vi "Read Controls.vi"(8 "Error In":errorcluster, 10 "Digital Input Task In":refnum<k21>, 11 "Analog Input Task In":refnum<k21>) -> (0 "Error Out":errorcluster, 1 "Octave Out":bool, 2 "Harmony Out":bool, 3 "Analog Input Task Out":refnum<k21>, 5 "Volume Out":dbl)   [LabVIEW 2020]
doc: "Read Controls.vi reads the voltage across the potentiometer and the state of the two digital buttons to determine the Volume double-precision floating-point value and the digital Harmony and Octave Boolean values."
uses:
  <vilib>/DAQmx/read.llb/DAQmx Read (Analog 1D DBL NChan 1Samp).vi
  <vilib>/DAQmx/read.llb/DAQmx Read (Digital 1D Bool 1Chan 1Samp).vi
  <vilib>/DAQmx/miscellaneous.llb/DAQmx Fill In Error Info.vi
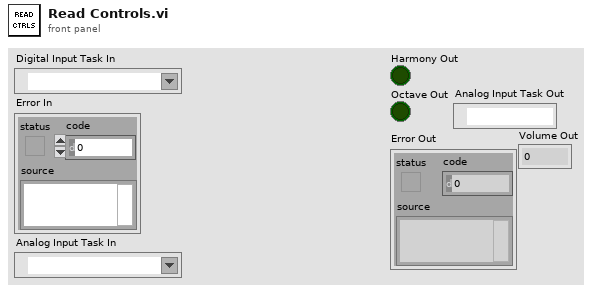
[diagram p1: front panel]
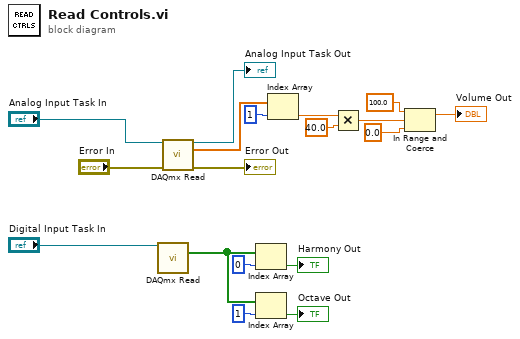
[diagram p0: block diagram]
diagram:
  n1 = call-poly <vilib>:"DAQmx Read.vi"("task/channels in"="Digital Input Task In") -> ("data"=w17:bool[])  [unwired: 12 in, 2 out]
  n2 = call-poly <vilib>:"DAQmx Read.vi"("task/channels in"="Analog Input Task In", "error in"="Error In") -> ("task out"=→"Analog Input Task Out":refnum<k21>, "data"=w13:dbl[], "error out"=→"Error Out":errorcluster)  [unwired: 11 in]
  n3 = Index Array(array=w17, index=0) -> (element=→"Harmony Out":bool)
  n4 = Index Array(array=w17, index=1) -> (element=→"Octave Out":bool)
  n5 = Index Array(array=w13, index=1) -> (element=w12:dbl)
  n6 = Multiply(x=w12, y=40.0) -> (x*y=w7:dbl)
  n7 = In Range and Coerce(upper limit=100.0, x=w7, lower limit=0.0) -> (coerced(x)=→"Volume Out":dbl)  [unwired: 1 out]
